vi "G#Object_New.vi"(0 "reference in":refnum<class "G#Object.lvclass">, 1 "object name":string, 4 "no registration? (F)":bool, 5 "error in (no error)":errorcluster, 6 "create method":T1=enum."Create or look up existing", 7 "user counter (T)?":bool=TRUE) -> (14 "reference out":refnum<class "G#Object.lvclass">, 17 "created new?":bool, 19 "error out":errorcluster)   [LabVIEW 2020, in "G#Object.lvclass"]
doc: "Creates a new object, but will also make it possible for the debugger process to create the object instead, this way, the debugger will own all of the queues and data value reference and single stepping of methods are possible."
uses:
  G#Object.lvclass
  utils/G#Object_CreateMethod.ctl
  G#Object.lvclass/G#Object.ctl
  utils/G#Object_EventType.ctl
  utils/G#Object_ObjectInfoType.ctl
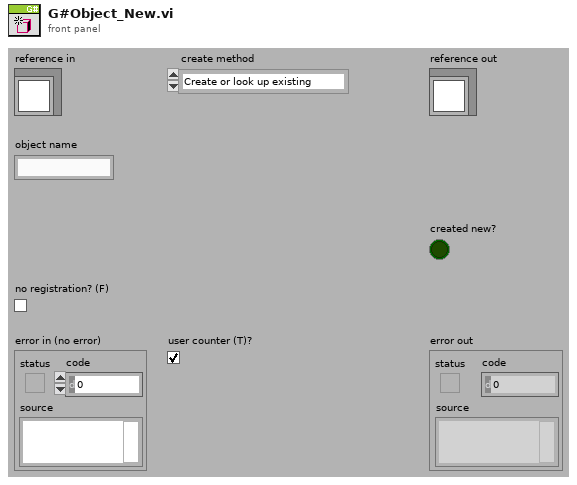
[diagram p1: front panel]
types:
  T1 = typedef "G#Object.lvclass/G#Object_CreateMethod.ctl" = enum16{"Create", "Create or look up existing", "Look up existing"}
  T2 = typedef "G#Object.lvclass/G#Object_ObjectInfoType.ctl" = cluster{"ObjectName":string, "ObjectID":u32, "Users":i32, "Counter":bool, "AttributeRefs":u32[], "FullClassName":string, "ClassName":string, "CreateMethod":T1, "GenericDestructorExists":bool, "Owner":string}
  T3 = typedef "G#Object.lvclass/G#Object_EventType.ctl" = enum16{"Created new", "Looked up existing", "Deleted", "Forced delete", "Not deleted", "Garbage collected", "Cleared", "User", "Error", "External create object", "External create class attributes", "Created class attributes", "Run constructor", "Run constructor done", "Run open method", "Run open method done"}
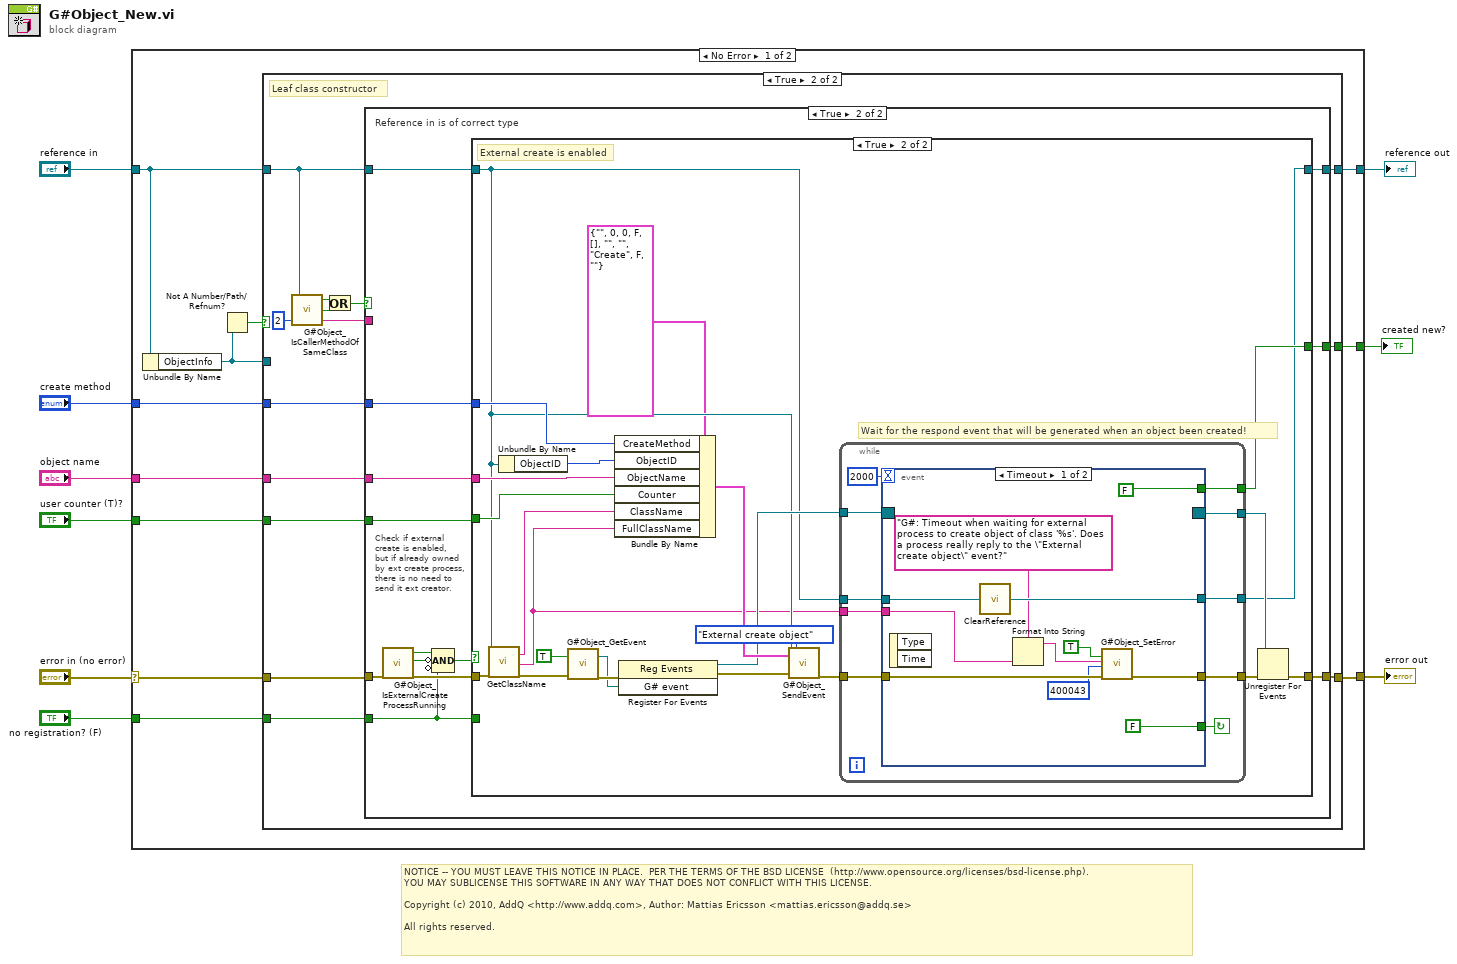
[diagram p0: block diagram]
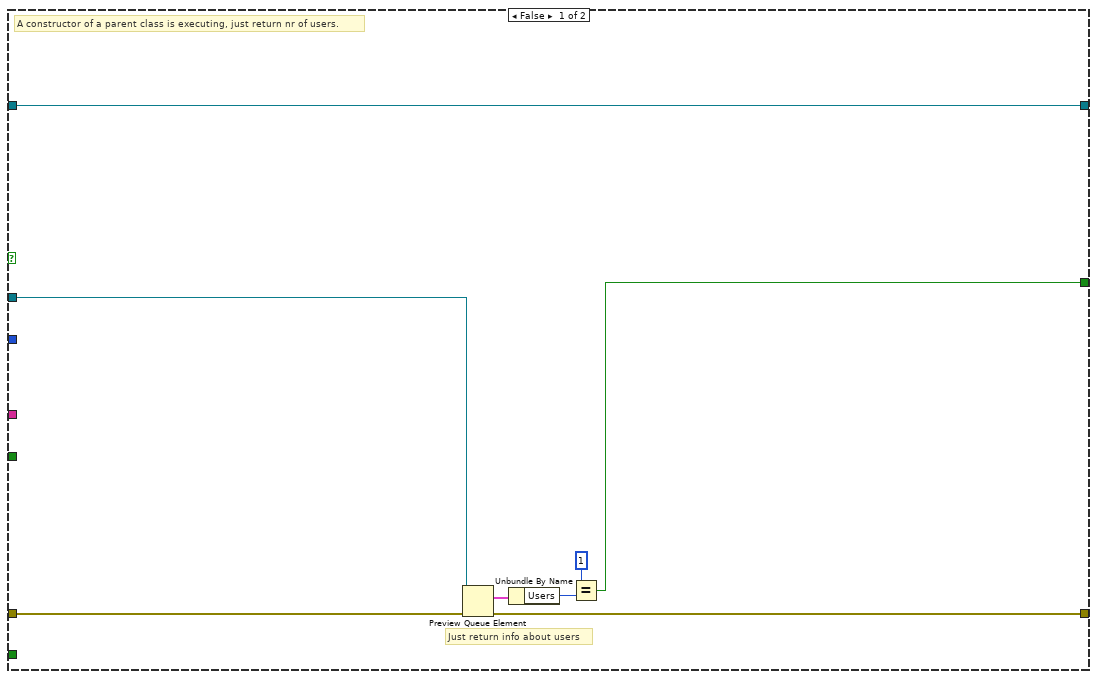
[diagram p2: hidden frame]
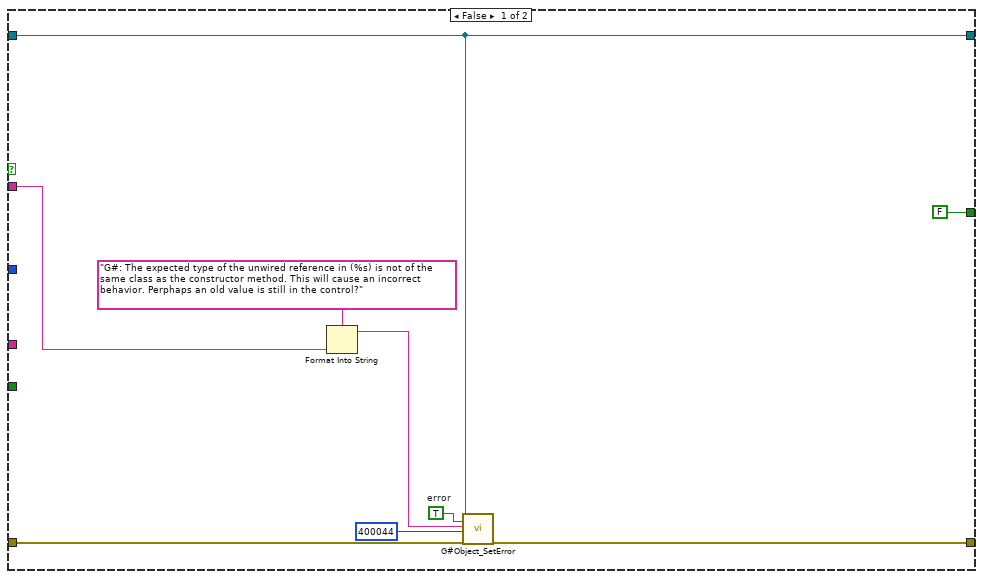
[diagram p3: hidden frame]
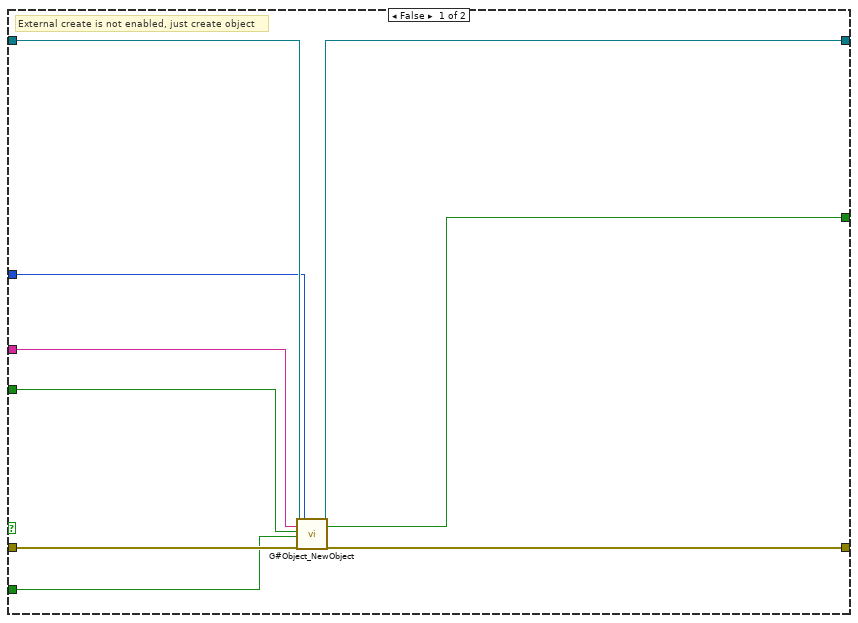
[diagram p4: hidden frame]
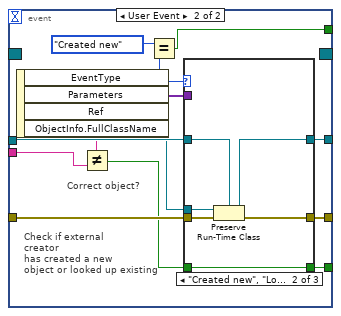
[diagram p5: hidden frame]
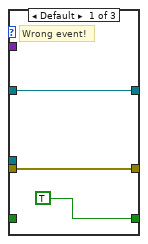
[diagram p6: hidden frame]
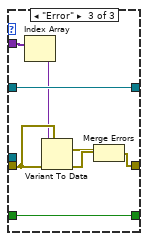
[diagram p7: hidden frame]
diagram:
  # "NOTICE -- YOU MUST LEAVE THIS NOTICE IN PLACE.  PER THE TERMS OF THE BSD LICENSE  (http://www.opensource.org/licenses/bsd-license.php).\nYOU MAY SUBLICENSE THIS SOFTWARE IN ANY WAY THAT DOES NOT CONFLICT WITH THIS LICENSE.\n\nCopyright (c) 2010, AddQ <http://www.addq.com>, Author: Mattias Ericsson <mattias.ericsson@addq.se>\n\nAll rights reserved."
  n1 = case shown="No Error" "error in (no error)" {
    selector: "error in (no error)" -> [w20 w149]
    tunnel: [w17 w149] -> w8
    tunnel: [w13 w148] -> w6
    tunnel: "reference in" -> [w14 w148]
    tunnel: "object name" -> [w19 _]
    tunnel: "user counter (T)?" -> [w18 _]
    tunnel: [w16 _] -> w3
    tunnel: "create method" -> [w12 _]
    tunnel: "no registration? (F)" -> [w11 _]
    frame No Error {
      n2 = Unbundle By Name(w14) -> ("ObjectInfo"=w15:refnum<queue>)
      n3 = Not A Number/Path/Refnum?(number/path/refnum=w15) -> (NaN/Path/Refnum?=w10:bool)
      n4 = case shown="True" w10 {
        tunnel: w20 -> [w28 w41]
        tunnel: w14 -> [w21 w33]
        tunnel: w19 -> [_ w38]
        tunnel: w18 -> [_ w39]
        tunnel: [w25 w40] -> w17
        tunnel: [w22 w42] -> w16
        tunnel: w15 -> [w27 _]
        tunnel: [w21 w37] -> w13
        tunnel: w12 -> [_ w36]
        tunnel: w11 -> [_ w35]
        frame False {
          # "A constructor of a parent class is executing, just return nr of users."
          # "Just return info about users"
          n5 = Preview Queue Element(queue=w27, error in (no error)=w28) -> (element=w26:T2, error out=w25:errorcluster)  [unwired: 1 in, 2 out]
          n6 = Unbundle By Name(w26) -> ("Users"=w24:i32)
          n7 = Equal?(x=1, y=w24) -> (x = y?=w22:bool)
        }
        frame True {
          # "Leaf class constructor"
          n8 = call "G#Object_IsCallerMethodOfSameClass.vi"("call depth (1)"=2 ("call depth"), "reference in"=w33) -> ("reference full class name"=w32:string, "is caller of G#Object?"=w29:bool, "is of same class?"=w31:bool)  [unwired: 1 in]
          n9 = Or(x=w31, y=w29) -> (x .or. y?=w30:bool)
          n10 = case shown="True" w30 {
            tunnel: [FALSE w58] -> w42
            tunnel: w41 -> [w50 w57]
            tunnel: [w48 w64] -> w40
            tunnel: w39 -> [_ w63]
            tunnel: w38 -> [_ w62]
            tunnel: [w49 w61] -> w37
            tunnel: w36 -> [_ w60]
            tunnel: w35 -> [_ w52]
            tunnel: w33 -> [w49 w59]
            tunnel: w32 -> [w46 _]
            frame False {
              w44 = TRUE  # error
              n11 = Format Into String(format string="G#: The expected type of the unwired reference in (%s) is not of the same class as the constructor method. This will cause an incorrect behavior. Perphaps an old value is still in the control?", w46) -> (resulting string=w45:string)  [unwired: 2 in, 1 out]
              n12 = call "G#Object_SetError.vi"("reference in"=w49, "error (F)"=w44, "source"=w45, "code"=400044, "error in (no error)"=w50) -> ("error out"=w48:errorcluster)  [unwired: 14 in]
            }
            frame True {
              # "Check if external\ncreate is enabled,\nbut if already owned\nby ext create process,\nthere is no need to\nsend it ext creator."
              # "Reference in is of correct type"
              n13 = call "G#Object_IsExternalCreateProcessRunning.vi"("error in (no error)"=w57) -> ("external create enabled?"=w55:bool, "owned by external process?"=w54:bool, "error out"=w56:errorcluster)  [unwired: 15 in, 1 out]
              n14 = Compound Arithmetic op=AND(w55, invert w54, invert w52) -> (w53:bool)
              n15 = case shown="True" w53 {
                tunnel: w56 -> [w73 w81]
                tunnel: [w72 w83] -> w64
                tunnel: w59 -> [w71 w77]
                tunnel: [w70 w78] -> w61
                tunnel: w60 -> [w69 w82]
                tunnel: w62 -> [w68 w94]
                tunnel: w63 -> [w67 w92]
                tunnel: w52 -> [w66 _]
                tunnel: [w65 w79] -> w58
                frame False {
                  # "External create is not enabled, just create object"
                  n16 = call "G#Object_NewObject.vi"("reference in"=w71, "object name (\"\")"=w68, "user counter (T)"=w67, "no registration (F)"=w66, "error in (no error)"=w73, "create method"=w69) -> ("reference out"=w70:refnum<class "G#Object.lvclass">, "created new?"=w65:bool, "error out"=w72:errorcluster)  [unwired: 11 in]
                }
                frame True {
                  # "External create is enabled"
                  # "Wait for the respond event that will be generated when an object been created!"
                  n17 = call-dynamic "GetClassName.vi"("reference in"=w77, "error in (no error)"=w81) -> ("class name"=w74:string, "full class name"=w75:string, "error out"=w80:errorcluster)  [unwired: 13 in, 2 out]
                  n18 = Unbundle By Name(w77) -> ("ObjectID"=w93:u32)
                  n19 = call "G#Object_GetEvent.vi"("create if needed (T)"=TRUE ("create if needed"), "error in (no error)"=w80) -> ("G# event"=w87:refnum<user-event>, "error out"=w90:errorcluster)  [unwired: 13 in, 3 out]
                  n20 = Bundle By Name(cluster=T2 {"ObjectName"="", "ObjectID"=0, "Users"=0, "Counter"=FALSE, "AttributeRefs"=[], "FullClassName"="", "ClassName"="", "CreateMethod"=enum."Create", "GenericDestructorExists"=FALSE, "Owner"=""} ("ObjectInfo"), "CreateMethod"=w82, "ObjectID"=w93, "ObjectName"=w94, "Counter"=w92, "ClassName"=w74, "FullClassName"=w75) -> (w95:T2)
                  n21 = register-events(error in=w90, w87) -> (reference out=w86:refnum<event-registration>, error out=w89:errorcluster)  [unwired: 1 in]
                  n22 = call "G#Object_SendEvent.vi"("reference in"=w77, "object info extended"=w95, "error in (no error)"=w89, "G# event type"=G#Object_EventType."External create object") -> ("error out"=w88:errorcluster)  [unwired: 15 in]
                  n23 = while {
                    tunnel: w88 -> [w106]
                    tunnel: w86 -> [w105]
                    tunnel: [w104] -> w85
                    tunnel: [w103] -> w84
                    tunnel: [w101] -> w78
                    tunnel: w77 -> [w100]
                    tunnel: [w99] -> w79
                    tunnel: w75 -> [w98]
                    stop <- w102 continue-if-true
                    n24 = event shown="[0] Timeout" {
                      selector: w105 -> [_ _]
                      dyn-events: [_ _] -> w104
                      timeout: 2000 ("y") -> [_ _]
                      tunnel: w106 -> [w114 w127]
                      tunnel: [w113 w126] -> w103
                      tunnel: [FALSE w125] -> w102
                      tunnel: [w117 w128] -> w101
                      tunnel: w100 -> [w116 w130]
                      tunnel: [FALSE w122] -> w99
                      tunnel: w98 -> [w111 w120]
                      event Timeout {
                        n25 = event-data() -> ()  [unwired: 1 in, 2 out]
                        n26 = call-dynamic "ClearReference.vi"("reference in"=w116) -> ("reference out"=w117:refnum<class "G#Object.lvclass">)
                        n27 = Format Into String(format string="G#: Timeout when waiting for external process to create object of class '%s'. Does a process really reply to the \"External create object\" event?", w111) -> (resulting string=w110:string)  [unwired: 2 in, 1 out]
                        n28 = call "G#Object_SetError.vi"("error (F)"=TRUE ("error"), "source"=w110, "code"=400043, "error in (no error)"=w114) -> ("error out"=w113:errorcluster)  [unwired: 15 in]
                      }
                      event User Event {
                        # "Correct object?"
                        # "Check if external\ncreator\nhas created a new\nobject or looked up existing"
                        n29 = event-data() -> ("EventType"=w124:T3, "Parameters"=w118:variant[], "Ref"=w129:refnum<class "G#Object.lvclass">, "ObjectInfo.FullClassName"=w121:string)  [unwired: 1 in]
                        n30 = Not Equal?(x=w121, y=w120) -> (x != y?=w119:bool)
                        n31 = Equal?(x=G#Object_EventType."Created new" ("EventType"), y=w124) -> (x = y?=w122:bool)
                        n32 = case shown="\"Created new\", \"Looked up existing\"" w124 {
                          tunnel: w130 -> [w132 w139 w147]
                          tunnel: w129 -> [_ w138 _]
                          tunnel: [w132 w137 w147] -> w128
                          tunnel: w127 -> [w133 w136 w146]
                          tunnel: [w133 w135 w144] -> w126
                          tunnel: [TRUE w134 w140] -> w125
                          tunnel: w119 -> [_ w134 w140]
                          tunnel: w118 -> [_ _ w145]
                          frame Default {
                            # "Wrong event!"
                          }
                          frame "Created new", "Looked up existing" {
                            n33 = Preserve Run-Time Class(object in=w138, error in=w136, 2:w139) -> (object out=w137:refnum<class "G#Object.lvclass">, error out=w135:errorcluster)
                          }
                          frame "Error" {
                            n34 = Index Array(array=w145) -> (element=w141:variant)  [unwired: 1 in]
                            n35 = Variant To Data(error in=w146, type=w146, Variant=w141) -> (data=w142:errorcluster, error out=w143:errorcluster)
                            n36 = Merge Errors(w142, w143) -> (w144:errorcluster)
                          }
                        }
                      }
                    }
                  }
                  n37 = Unregister For Events(event registration refnum=w85, error in=w84) -> (error out=w83:errorcluster)
                }
              }
            }
          }
        }
      }
    }
    frame Error {
    }
  }
  "error out" <- w8
  "reference out" <- w6
  "created new?" <- w3
